vi "cRIO FTP dirlist.vi"(8 "Fehler (in)":errorcluster caption="Fehlerkonstante", 11 "dir":string) -> (0 "Fehler (out)":errorcluster caption="Fehlerkonstante", 3 "dir list":string[](array[string]))   [LabVIEW 2015, in "SysLog.lvlib"]
uses:
  SysLog.lvlib
  <vilib>/FTP/NI_FTP.lvlib
  <vilib>/WebDAVClient/NI_WebDAV.lvlib
panel:
  out "reply string":string
  out "reply code":i32
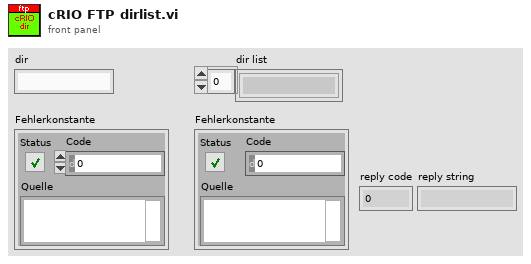
[diagram p1: front panel]
types:
  T1 = typedef "NI_FTP.lvlib/FTP Session.ctl" = refnum<k5>
  T2 = typedef "NI_FTP.lvlib/FTP File Info.ctl" = cluster{"type":enum16{"unknown", "file", "dir", "link"}, "permissions":string, "owner":string, "group":string, "size":i32, "date":string, "name":string, "link name":string}
  T3 = typedef "NI_WebDAV.lvlib/SessionHandle.ctl" = refnum<k1>
  T4 = typedef "NI_WebDAV.lvlib/FileInfo.ctl" = cluster{"type":string, "size":u64, "last modification":timestamp, "display name":string, "uri":string}
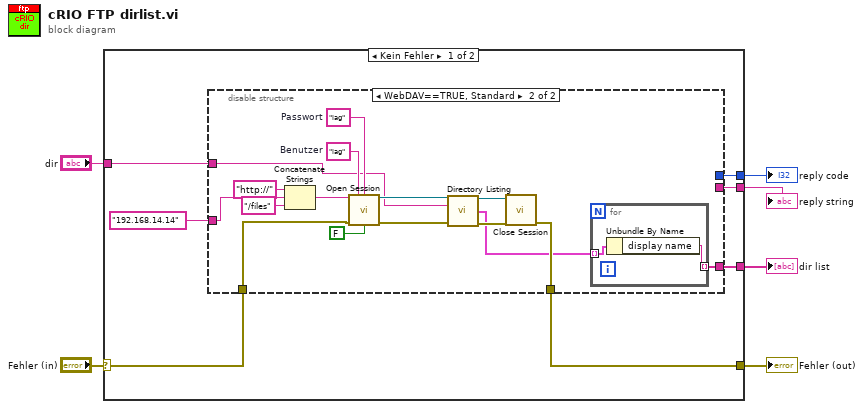
[diagram p0: block diagram]
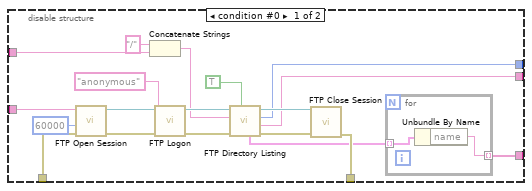
[diagram p2: hidden frame]
diagram:
  n1 = case shown="Kein Fehler" "Fehler (in)" {
    selector: "Fehler (in)" -> [w13 w53]
    tunnel: [w12 w53] -> w5
    tunnel: [w11 _] -> w1
    tunnel: "dir" -> [w10 _]
    tunnel: [w8 _] -> w3
    tunnel: [w7 _] -> w2
    frame No Error {
      n2 = disable-structure shown="WebDAV==TRUE, Standard" {
        disable-tunnel: w13 -> [w26 w40]
        disable-tunnel: [w25 w39] -> w12
        disable-tunnel: [w16 w35] -> w11
        disable-tunnel: w10 -> [w24 w37]
        disable-tunnel: "192.168.14.14" ("address") -> [w23 w38]
        disable-tunnel: [w21 _] -> w8
        disable-tunnel: [w20 _] -> w7
        frame condition #0 {
          n3 = call <vilib>:"FTP Open Session.vi"("error in (no error)"=w26, "timeout ms (60000)"=60000, "address"=w23) -> ("error out"=w30:errorcluster, "ftp session"=w32:T1)  [unwired: 5 in, 2 out]
          n4 = Concatenate Strings("/" ("String"), w24) -> (w15:string)
          n5 = call <vilib>:"FTP Logon.vi"("error in (no error)"=w30, "user"="anonymous", "ftp session"=w32) -> ("error out"=w29:errorcluster, "ftp session out"=w31:T1)  [unwired: 5 in, 2 out]
          n6 = call <vilib>:"FTP Directory Listing.vi"("active (T)"=TRUE, "error in (no error)"=w29, "directory path"=w15, "ftp session"=w31) -> ("error out"=w28:errorcluster, "reply string"=w20:string, "reply code"=w21:i32, "ftp session out"=w27:T1, "dir list"=w17:T2[])  [unwired: 3 in]
          n7 = call <vilib>:"FTP Close Session.vi"("error in (no error)"=w28, "ftp session"=w27) -> ("error out"=w25:errorcluster)  [unwired: 6 in, 3 out]
          n8 = for {
            tunnel: w17 -> [w34] mode=indexing
            tunnel: [w33] -> w16 mode=indexing
            n9 = Unbundle By Name(w34) -> ("name"=w33:string)
          }
        }
        frame condition #1 (active) {
          w47 = "iag"  # Passwort
          w46 = "iag"  # Benutzer
          n10 = Concatenate Strings("http://" ("String"), w38, "/files" ("String")) -> (w45:string)
          n11 = call <vilib>:"Open Session.vi"("host uri prefix"=w45, "username"=w46, "password"=w47, "error in (no error)"=w40, "verify server?"=FALSE) -> ("session handle out"=w49:T3, "error out"=w50:errorcluster)  [unwired: 9 in]
          n12 = call <vilib>:"Directory Listing.vi"("session handle"=w49, "relative uri"=w37, "error in (no error)"=w50) -> ("session handle out"=w42:T3, "file list"=w36:T4[], "error out"=w41:errorcluster)  [unwired: 9 in, 1 out]
          n13 = call <vilib>:"Close Session.vi"("session handle"=w42, "error in (no error)"=w41) -> ("error out"=w39:errorcluster)  [unwired: 13 in]
          n14 = for {
            tunnel: w36 -> [w52] mode=indexing
            tunnel: [w51] -> w35 mode=indexing
            n15 = Unbundle By Name(w52) -> ("display name"=w51:string)
          }
        }
      }
    }
    frame Error {
    }
  }
  "Fehler (out)" <- w5
  "reply code" <- w3
  "reply string" <- w2
  "dir list" <- w1
